vi "AMX-电源尾反面漏线检测.vi"(8 "error in (no error)":errorcluster caption="错误输入（无错误）", 9 "UI电源线正面漏线参数":T4={"Rectangle"={"Left"=0, "Top"=0, "Right"=0, "Bottom"=0, "Rotation"=0.0}, "模板路径"=path "C:/Users/delluser001/Desktop/PowerLine Inspect System/Source Code/Template Program/potteryTemplete/Color.png", "Match Mode "=0, "Minimum Match Score "=800.0, "Number of Matches Requested"=1, "Rotation Angle Ranges (degrees)"=[{"Min"=-180.0, "Max"=180.0}], "Color Sensitivity "=0, "Match Offset"={"X"=0.0, "Y"=0.0}, "Color Score Weight "=500.0, "Search Strategy "=0, "Subpixel Accuracy "=FALSE, "Range (Threshold 1)"={"Lower value"=148.0, "Upper value"=255.0}} {"Search Strategy" items=["Conservative", "Balance", "Aggressive", "Very Aggressive"]; "Color Sensitivity" items=["Low Sensitivity", "Medium Sensitivity", "High Sensitivity"]; "Match Mode" items=["Shift Invariant", "Rotation Invariant"]; "Rectangle"."Rotation" format="%.2f"; "Rectangle"."Left" scale=0.0..1024.0; "Rectangle"."Right" scale=0.0..1024.0}, 10 "电源线正面标签1基础参数":T2={"IsNorImage"=TRUE, "Exposure Values"=100289, "ImagePath"=path "C:/Users/hedongpo/Desktop/514-hdp/Alignment Assemble System/Test Picture/B/3.bmp"} caption="参数界面" {"Exposure Values" scale=0.0..200000.0}, 11 "Image in":T1(plugin-control)) -> (0 "error out":errorcluster caption="错误输出", 3 "Image out":T1(plugin-control), 5 "x = 0?":bool)   [LabVIEW 2017]
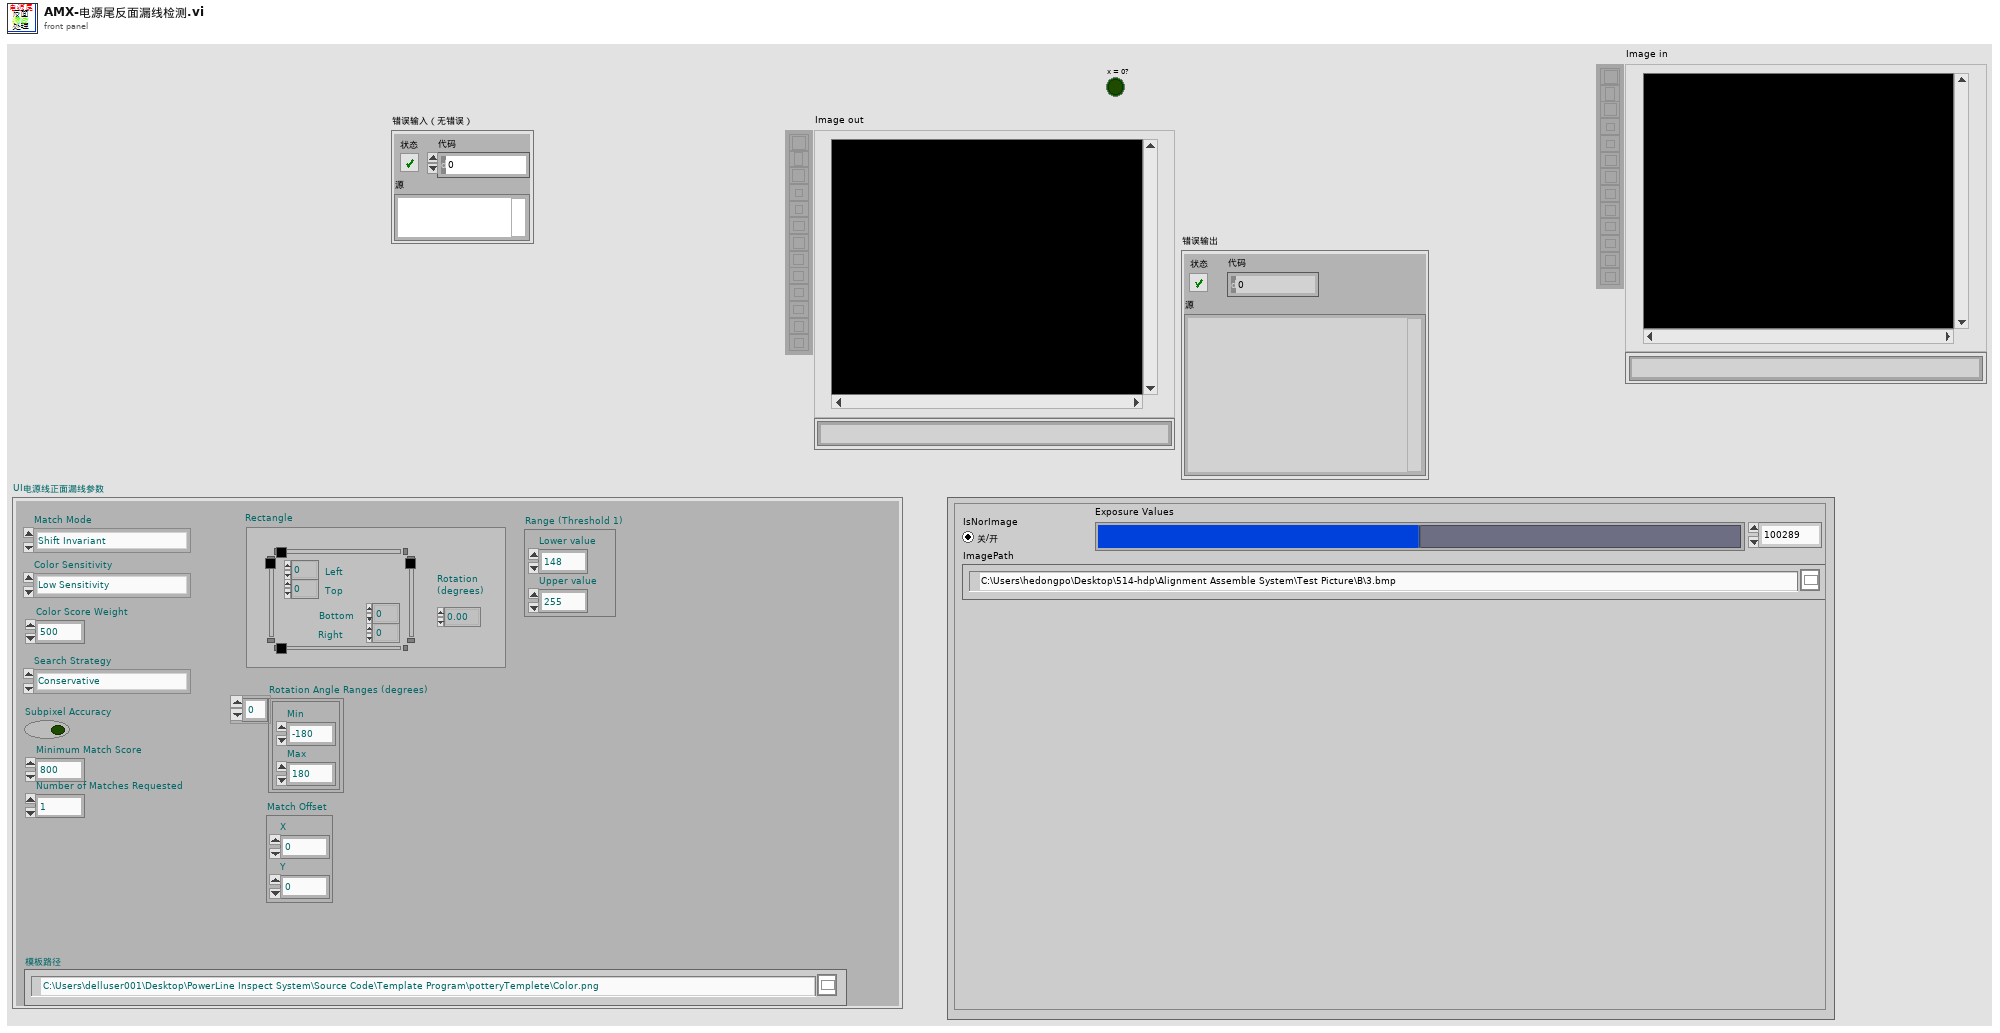
[diagram p1: front panel]
types:
  T1 = typedef "IMAQ Image.ctl" = refnum<image>
  T2 = cluster{"IsNorImage":bool, "Exposure Values":u32, "ImagePath":path}
  T3 = typedef "IMAQ Rectangle" = cluster{"Left":i32, "Top":i32, "Right":i32, "Bottom":i32, "Rotation":dbl}
  T4 = cluster{"Rectangle":T3, "模板路径":path, "Match Mode ":u32, "Minimum Match Score ":sgl, "Number of Matches Requested":i32, "Rotation Angle Ranges (degrees)":cluster{"Min":sgl, "Max":sgl}[], "Color Sensitivity ":u32, "Match Offset":cluster{"X":sgl, "Y":sgl}, "Color Score Weight ":sgl, "Search Strategy ":u32, "Subpixel Accuracy ":bool, "Range (Threshold 1)":cluster{"Lower value":sgl, "Upper value":sgl}}
  T5 = typedef "Image Type" = u32
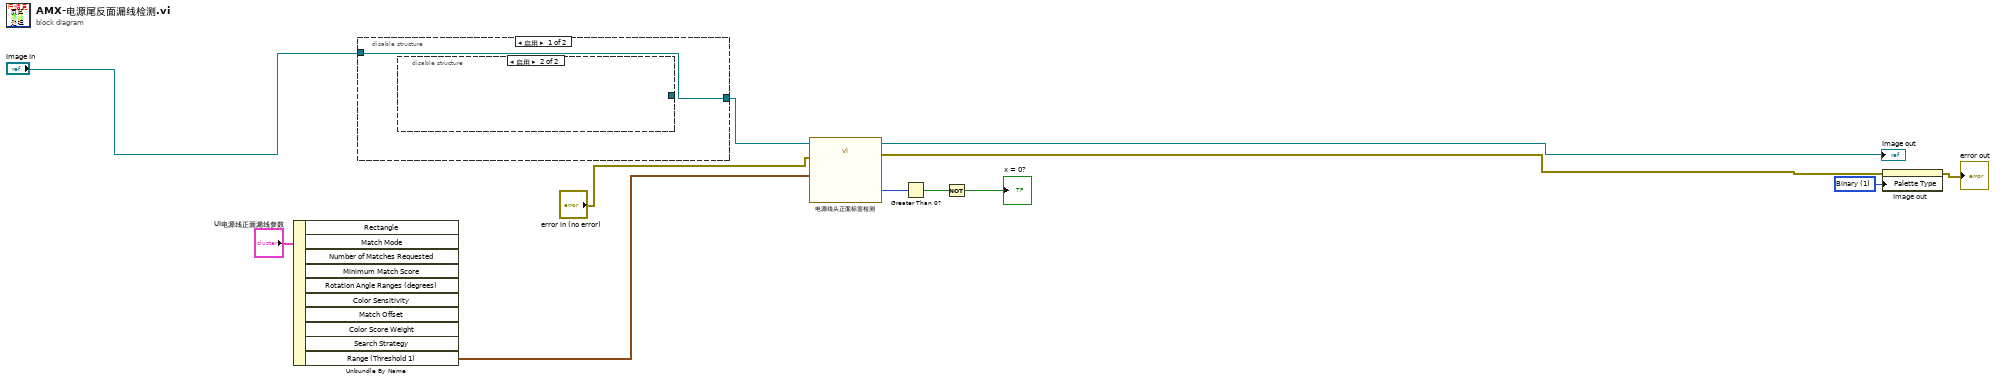
[diagram p0: block diagram]
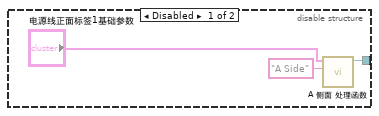
[diagram p2: hidden frame]
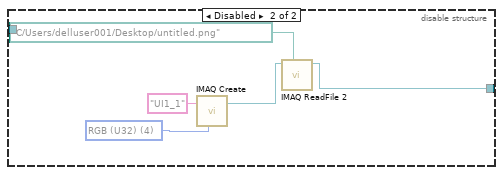
[diagram p3: hidden frame]
diagram:
  w11 = u32 1 items=["Grayscale", "Binary", "Gradient", "Rainbow", "Temperature", "User Defined", "Binary 16 Bit", "Gradient 16 Bit", "Rainbow 16 Bit", "Temperature 16 Bit", "User Defined 16 Bit"] ("Palette:Palette Type")
  n1 = Unbundle By Name("UI电源线正面漏线参数") -> ("Range (Threshold 1)"=w7:cluster{"Lower value":sgl, "Upper value":sgl})  [unwired: 9 out]
  n2 = disable-structure shown="启用" {
    disable-tunnel: [w13 w17] -> w9
    disable-tunnel: "Image in" -> [w13 _]
    frame Enabled {
      n3 = disable-structure shown="启用" {
        disable-tunnel: [w14 _] -> _
        frame Disabled {
          n4 = call "A 侧面 处理函数.vi"("Image Name"="A Side", "ParamsUI"="电源线正面标签1基础参数") -> ("Image out"=w14:T1)  [unwired: 6 in, 3 out]
        }
        frame Enabled {
        }
      }
    }
    frame Disabled {
      w20 = T5 4 items=["Grayscale (U8)", "Grayscale (I16)", "Grayscale (SGL)", "Complex (CSG)", "RGB (U32)", "HSL (U32)", "RGB (U64)", "Grayscale (U16)"] ("Image Type")
      n5 = call "IMAQ Create"("Image Name"="UI1_1", "Image Type"=w20) -> ("New Image"=w19:T1)  [unwired: 3 in, 1 out]
      n6 = call "IMAQ ReadFile 2"("File Path"=path "C:/Users/delluser001/Desktop/untitled.png", "Image"=w19) -> ("Image Out"=w17:T1)  [unwired: 5 in, 4 out]
    }
  }
  n7 = call "电源线头正面标签检测"("Image In"=w9, "error in"="error in (no error)", "Range (Threshold 1)"=w7) -> ("Image Out"=→"Image out":T1, "error out"=w5:errorcluster, "Number of Particles (Particle Analysis 1)"=w4:i32)  [unwired: 22 in]
  n8 = Greater Than 0?(x=w4) -> (x > 0?=w3:bool)
  n9 = Not(x=w3) -> (.not. x?=→"x = 0?":bool)
  n10 = property on="Image out" class="ImageControl"(error in=w5, "Palette Type"=w11) -> (error out=→"error out":errorcluster)  [unwired: 1 in, 1 out]
